vi "ControlsArbiter.vi"(0 "Manual Setpoints":T4, 5 "Dont Flip Setpoints":T4, 7 "Get out of Irons Setpoints":T4, 9 "Get to Goal Setpoints":T4, 11 "Default Setpoints":T4) -> (8 "Final Setpoints":T1)   [LabVIEW 2011]
uses:
  2 Typedefs/setpoints to arbiter.ctl
  2 Typedefs/setpoints to boat.ctl
  2 Typedefs/sail setpt.ctl
  2 Typedefs/rudder angle.ctl
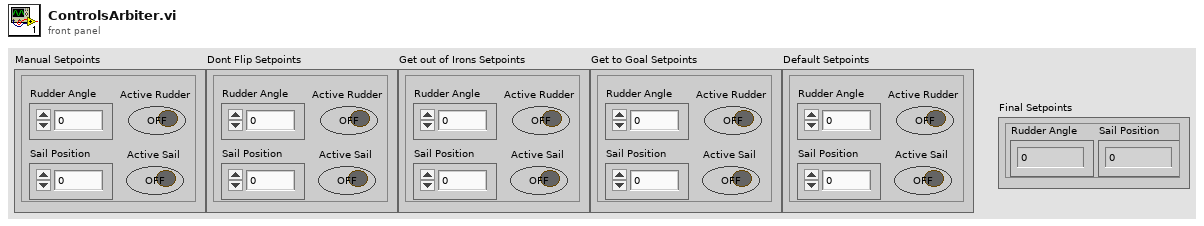
[diagram p1: front panel]
types:
  T1 = typedef "setpoints to boat.ctl" = cluster{"Sail Position":T2, "Rudder Angle":T3}
  T2 = typedef "sail setpt.ctl" = dbl
  T3 = typedef "rudder angle.ctl" = dbl
  T4 = typedef "setpoints to arbiter.ctl" = cluster{"Rudder Angle":dbl, "Sail Position":dbl, "Active Rudder":bool, "Active Sail":bool}
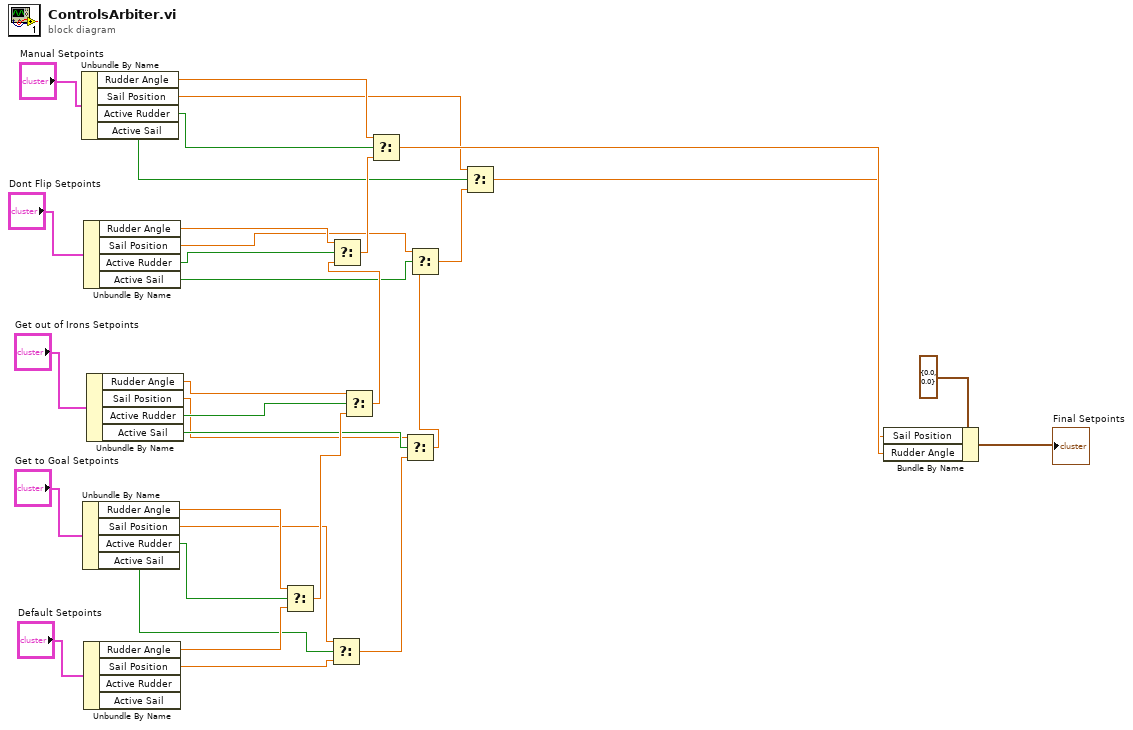
[diagram p0: block diagram]
diagram:
  n1 = Unbundle By Name("Manual Setpoints") -> ("Rudder Angle"=w22:dbl, "Sail Position"=w13:dbl, "Active Rudder"=w21:bool, "Active Sail"=w14:bool)
  n2 = Unbundle By Name("Get to Goal Setpoints") -> ("Rudder Angle"=w27:dbl, "Sail Position"=w5:dbl, "Active Rudder"=w28:bool, "Active Sail"=w4:bool)
  n3 = Unbundle By Name("Dont Flip Setpoints") -> ("Rudder Angle"=w19:dbl, "Sail Position"=w11:dbl, "Active Rudder"=w18:bool, "Active Sail"=w10:bool)
  n4 = Unbundle By Name("Default Setpoints") -> ("Rudder Angle"=w26:dbl, "Sail Position"=w3:dbl)  [unwired: 2 out]
  n5 = Unbundle By Name("Get out of Irons Setpoints") -> ("Rudder Angle"=w23:dbl, "Sail Position"=w7:dbl, "Active Rudder"=w24:bool, "Active Sail"=w8:bool)
  n6 = Select(t=w27, s=w28, f=w26) -> (s? t:f=w25:dbl)
  n7 = Select(t=w5, s=w4, f=w3) -> (s? t:f=w6:dbl)
  n8 = Select(t=w23, s=w24, f=w25) -> (s? t:f=w17:dbl)
  n9 = Select(t=w19, s=w18, f=w17) -> (s? t:f=w20:dbl)
  n10 = Select(t=w22, s=w21, f=w20) -> (s? t:f=w15:dbl)
  n11 = Select(t=w7, s=w8, f=w6) -> (s? t:f=w9:dbl)
  n12 = Select(t=w11, s=w10, f=w9) -> (s? t:f=w12:dbl)
  n13 = Select(t=w13, s=w14, f=w12) -> (s? t:f=w2:dbl)
  n14 = Bundle By Name(cluster=T1 {"Sail Position"=0.0, "Rudder Angle"=0.0} ("Setpoints"), "Sail Position"=w2, "Rudder Angle"=w15) -> (→"Final Setpoints":T1)
